vi "Display.vi"(7 "Action":u16(ring) items=["Read", "Initialize"], 9 "displayed matrix":u8[][](array[numeric])=array600x792[475200 elements]) -> (0 "Read action":u16)   [LabVIEW 2014]
panel:
  in  "Display Width (px)":i32=3840
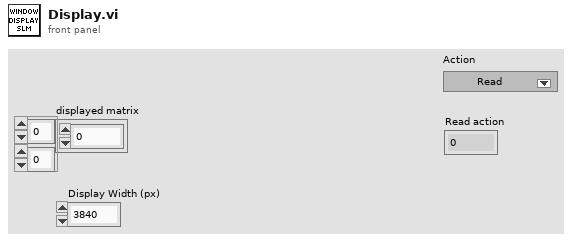
[diagram p1: front panel]
types:
  T1 = typedef "IMAQ Image.ctl" = refnum<image>
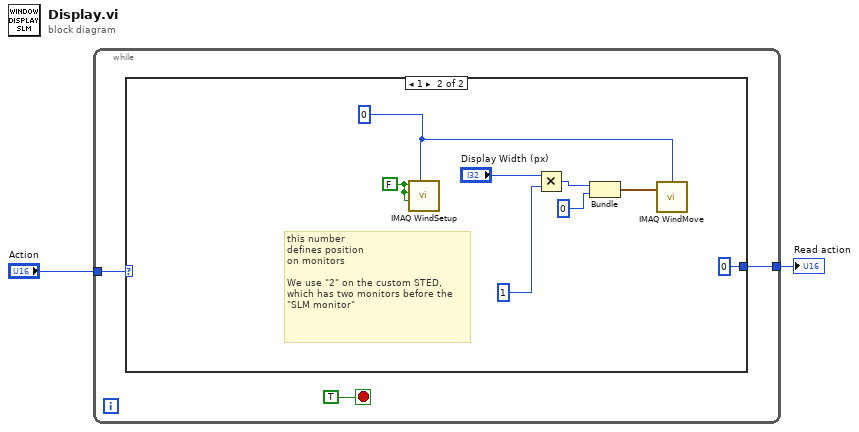
[diagram p0: block diagram]
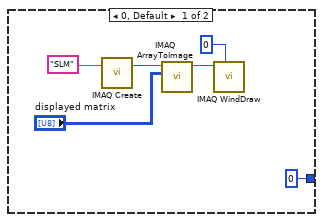
[diagram p2: hidden frame]
diagram:
  n1 = while {
    tunnel: "Action" -> [w4]
    tunnel: [w3] -> w2
    stop <- TRUE stop-if-true
    n2 = case shown="1" w4 {
      tunnel: [u16 0 ("Action 2") u16 0 ("Action 2")] -> w3
      frame 0, Default {
        n3 = call "IMAQ Create"("Image Name"="SLM") -> ("New Image"=w10:T1)  [unwired: 3 in, 2 out]
        n4 = call "IMAQ ArrayToImage"("Image Pixels (U8)"="displayed matrix", "Image"=w10) -> ("Image Out"=w11:T1)  [unwired: 4 in, 5 out]
        n5 = call "IMAQ WindDraw"("Window Number (0...15)"=0 ("number"), "Image"=w11) -> ()  [unwired: 4 in, 6 out]
      }
      frame 1 {
        w12 = 0
        w19 = FALSE ("Window can grow? (Yes)")
        # "this number\ndefines position\non monitors\n\nWe use \"2\" on the custom STED, which has two monitors before the \"SLM monitor\""
        n6 = call "IMAQ WindSetup"("Window Number (0...15)"=w12, "Window has title bar? (Yes)"=w19, "Window can close? (Yes)"=w19, "Window can grow? (Yes)"=w19) -> ()  [unwired: 3 in, 5 out]
        n7 = Multiply(x="Display Width (px)", y=1) -> (x*y=w16:i32)
        n8 = Bundle(w16, 0) -> (w17:cluster{i32, i32})  [unwired: 1 out]
        n9 = call "IMAQ WindMove"("Window Number (0...15)"=w12, "Coordinates (screen)"=w17) -> ()  [unwired: 2 in, 3 out]
      }
    }
  }
  "Read action" <- w2
